vi "Get Displays.vi"(1 "GPIB addess":string="17", 3 "Read C?":bool) -> (9 "A Overflow":bool, 11 "B Overflow":bool, 14 "display A":dbl format="%.3e", 15 "display B":dbl format="%.3e", 16 "display C":dbl format="%.3e", 17 "Function A":T2(ring), 18 "Function B":T1(ring), 19 "Unit C":enum16{"kHz", "V", "mA", "Reference Data"}(ring))   [LabVIEW 2009, in "HP4192A IA.lvclass"]
uses:
  HP4192A IA.lvclass
panel:
  out "Debug String 2":string
  out "Debug String":string
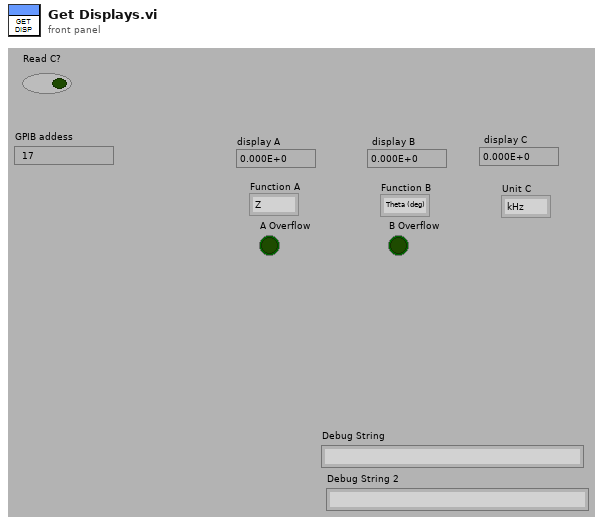
[diagram p1: front panel]
types:
  T1 = enum16{"Theta (deg)", "Theta (rad)", "X", "B", "Q", "D", "R", "G", "GROUP DELAY", "Unmeasure"}
  T2 = enum16{"Z", "Y", "R", "G", "L (Series)", "L (Parallel)", "C (Series)", "C (Parallel)", "B - A (dB)", "A (dBV)", "B (dBV)", "A (dBm)", "B (dBm)"}
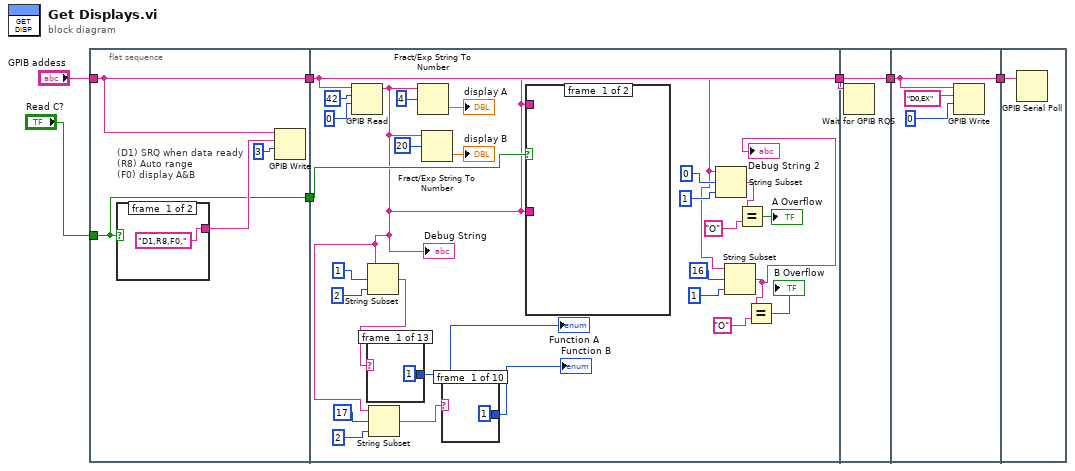
[diagram p0: block diagram]
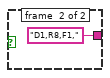
[diagram p2: hidden frame]
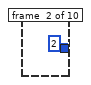
[diagram p3: hidden frame]
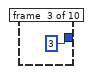
[diagram p4: hidden frame]
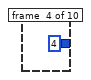
[diagram p5: hidden frame]
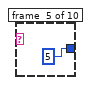
[diagram p6: hidden frame]
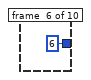
[diagram p7: hidden frame]
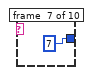
[diagram p8: hidden frame]
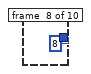
[diagram p9: hidden frame]
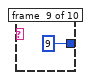
[diagram p10: hidden frame]
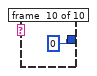
[diagram p11: hidden frame]
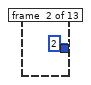
[diagram p12: hidden frame]
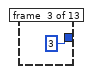
[diagram p13: hidden frame]
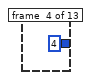
[diagram p14: hidden frame]
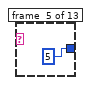
[diagram p15: hidden frame]
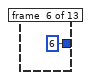
[diagram p16: hidden frame]
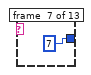
[diagram p17: hidden frame]
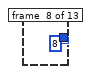
[diagram p18: hidden frame]
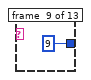
[diagram p19: hidden frame]
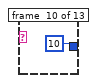
[diagram p20: hidden frame]
diagram:
  n1 = flat-sequence {
    tunnel: "GPIB addess" -> [w9]
    tunnel: [w9] -> w6
    tunnel: "Read C?" -> [w8]
    tunnel: [w8] -> w1
    tunnel: w6 -> [w34]
    tunnel: [w34] -> w5
    tunnel: w1 -> [w33]
    tunnel: w5 -> [w76]
    tunnel: [w76] -> w4
    tunnel: w4 -> [w79]
    tunnel: [w79] -> w3
    tunnel: w3 -> [w80]
    frame #0 {
      # "(D1) SRQ when data ready\n(R8) Auto range\n(F0) display A&B"
      n2 = case shown="True" w8 {
        tunnel: ["D1,R8,F0," "D1,R8,F1,"] -> w10
        frame #0 {
        }
        frame #1 {
        }
      }
      n3 = GPIB Write(0:w9, 1:w10, 2:3) -> ()  [unwired: 2 in, 2 out]
    }
    frame #1 {
      n4 = GPIB Read(0:w34, 1:42, 2:0) -> (5:w15:string)  [unwired: 2 in, 2 out]
      "Debug String" <- w15
      n5 = String Subset(string=w15, offset (0)=1, length (rest)=2) -> (substring=w29:string)
      n6 = case shown="\"ZF\"" w29 {
        tunnel: [1 2 3 4 5 6 7 8 9 10 11 12 0] -> w30
        frame #0 {
        }
        frame #1 {
        }
        frame #2 {
        }
        frame #3 {
        }
        frame #4 {
        }
        frame #5 {
        }
        frame #6 {
        }
        frame #7 {
        }
        frame #8 {
        }
        frame #9 {
        }
        frame #10 {
        }
        frame #11 {
        }
        frame #12 {
        }
      }
      "Function A" <- w30
      n7 = String Subset(string=w15, offset (0)=17, length (rest)=2) -> (substring=w25:string)
      n8 = Fract/Exp String To Number(string=w15, offset=4) -> (number=→"display A":dbl)  [unwired: 2 in, 1 out]
      n9 = Fract/Exp String To Number(string=w15, offset=20) -> (number=→"display B":dbl)  [unwired: 2 in, 1 out]
      n10 = case shown="\"TD\", Default" w25 {
        tunnel: [1 2 3 4 5 6 7 8 9 0] -> w28
        frame #0 {
        }
        frame #1 {
        }
        frame #2 {
        }
        frame #3 {
        }
        frame #4 {
        }
        frame #5 {
        }
        frame #6 {
        }
        frame #7 {
        }
        frame #8 {
        }
        frame #9 {
        }
      }
      "Function B" <- w28
      n11 = case shown="True" w33 {
        tunnel: w15 -> [_ w70]
        tunnel: w15 -> [_ w66]
        frame #0 {
        }
        frame #1 {
          n12 = Fract/Exp String To Number(string=w70, offset=33) -> (number=→"display C":dbl)  [unwired: 2 in, 1 out]
          n13 = String Subset(string=w66, offset (0)=32, length (rest)=1) -> (substring=w64:string)
          n14 = case shown="\"R\"" w64 {
            tunnel: [1 2 3 0] -> w65
            frame #0 {
            }
            frame #1 {
            }
            frame #2 {
            }
            frame #3 {
            }
          }
          "Unit C" <- w65
        }
      }
      n15 = String Subset(string=w15, offset (0)=0, length (rest)=1) -> (substring=w21:string)
      n16 = String Subset(string=w15, offset (0)=16, length (rest)=1) -> (substring=w14:string)
      "Debug String 2" <- w14
      n17 = Equal?(x=w21, y="O") -> (x = y?=→"A Overflow":bool)
      n18 = Equal?(x=w14, y="O") -> (x = y?=→"B Overflow":bool)
    }
    frame #2 {
      n19 = Wait for GPIB RQS(4:w76) -> ()  [unwired: 2 in, 2 out]
    }
    frame #3 {
      n20 = GPIB Write(0:w79, 1:"D0,EX", 2:0) -> ()  [unwired: 2 in, 2 out]
    }
    frame #4 {
      n21 = GPIB Serial Poll(0:w80) -> ()  [unwired: 1 in, 3 out]
    }
  }
